vi "Get Core Message.vi"(8 "error in (no error)":errorcluster, 11 "Message":refnum<class "MSG.lvclass">) -> (0 "error out":errorcluster, 2 "Core Message":refnum<class "MSG.lvclass">, 3 "Message Envelope":refnum<class "MSG.lvclass">)   [LabVIEW 2011, in "Messenging.lvlib" / "MSG.lvclass"]
uses:
  MSG.lvclass
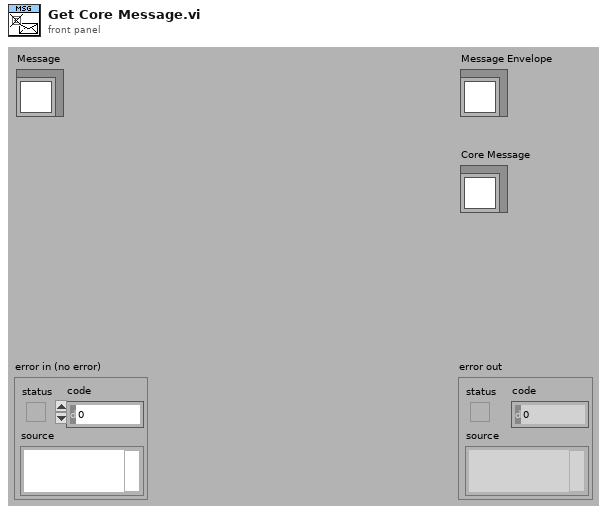
[diagram p1: front panel]
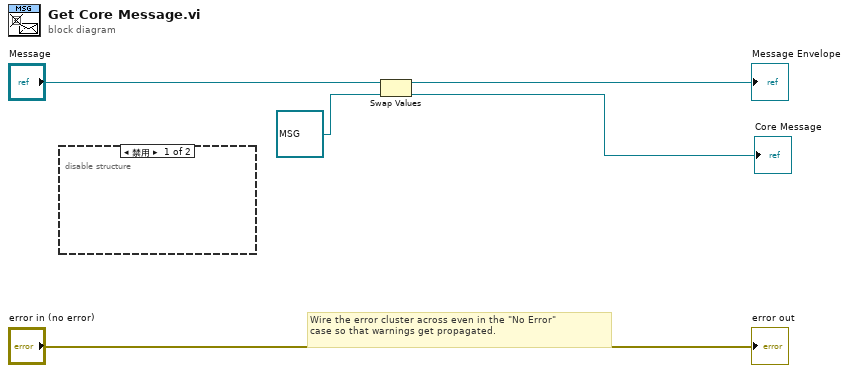
[diagram p0: block diagram]
diagram:
  # "Wire the error cluster across even in the \"No Error\"\ncase so that warnings get propagated."
  n1 = disable-structure shown="禁用" {
    frame Disabled {
    }
    frame Enabled {
    }
  }
  n2 = Swap Values(12:"Message", 14:refnum<class "MSG.lvclass"> refnum ("Message")) -> (1:→"Message Envelope":refnum<class "MSG.lvclass">, 3:→"Core Message":refnum<class "MSG.lvclass">)  [unwired: 1 out]
  "error out" <- "error in (no error)"
